vi "configuration_pv_subsystem.vi"() -> (3 "configuration_pv_subsystem":T1={"enable_mrc"=0, "hologram_composition"=1, "recording_indicator"=0, "video_stabilization"=0, "blank_protected"=0, "show_mesh"=0, "shared"=0, "_reserved_0"=0, "global_opacity"=0.9, "output_width"=0.0, "output_height"=0.0, "video_stabilization_length"=0, "hologram_perspective"=1, "_reserved_1"=0})   [LabVIEW 2023]
panel:
  in  "configuration_pv_subsystem":T1={"enable_mrc"=0, "hologram_composition"=1, "recording_indicator"=0, "video_stabilization"=0, "blank_protected"=0, "show_mesh"=0, "shared"=0, "_reserved_0"=0, "global_opacity"=0.9, "output_width"=0.0, "output_height"=0.0, "video_stabilization_length"=0, "hologram_perspective"=1, "_reserved_1"=0}
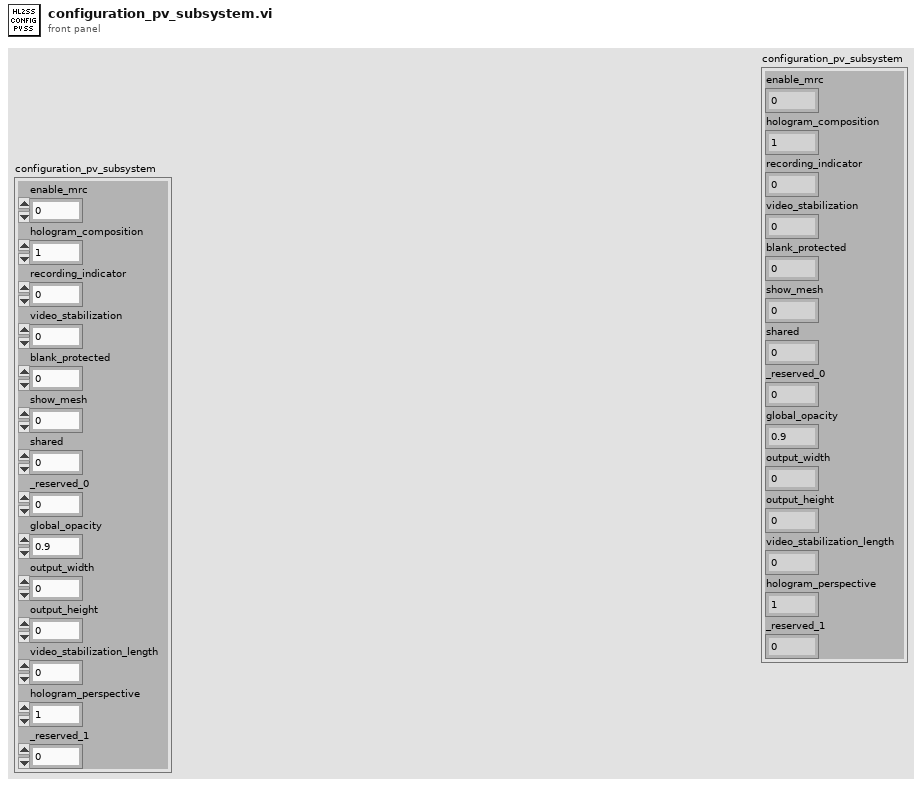
[diagram p1: front panel]
types:
  T1 = cluster{"enable_mrc":u8, "hologram_composition":u8, "recording_indicator":u8, "video_stabilization":u8, "blank_protected":u8, "show_mesh":u8, "shared":u8, "_reserved_0":u8, "global_opacity":sgl, "output_width":sgl, "output_height":sgl, "video_stabilization_length":u32, "hologram_perspective":u32, "_reserved_1":u32}
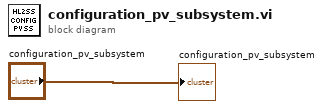
[diagram p0: block diagram]
diagram:
  "configuration_pv_subsystem" <- "configuration_pv_subsystem"
